vi "Coersion.vi"() -> ()   [LabVIEW 2011]
panel:
  out "In Range?":bool
  out "?":dbl
  in  "x":dbl
  in  "lower limit":dbl
  in  "upper limit":dbl
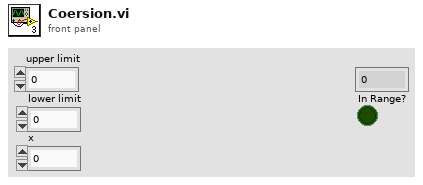
[diagram p1: front panel]
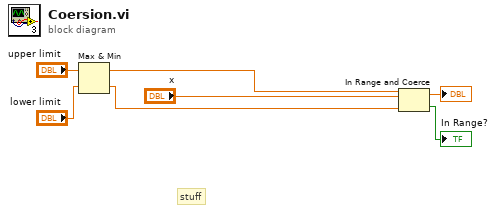
[diagram p0: block diagram]
diagram:
  # "stuff"
  n1 = Max & Min(x="upper limit", y="lower limit") -> (max(x,y)=w2:dbl, min(x,y)=w1:dbl)
  n2 = In Range and Coerce(upper limit=w2, x="x", lower limit=w1) -> (coerced(x)=→"?":dbl, In Range?=→"In Range?":bool)
